vi "FTW-Example-SLASD-Add Actor.vi"(0 "FTW-Example-SLASD In":refnum<class "FTW-Example-SLASD.lvclass">, 11 "error in (no error)":errorcluster) -> (4 "FTW-Example-SLASD Out":refnum<class "FTW-Example-SLASD.lvclass">, 15 "error out":errorcluster)   [LabVIEW 2013, in "FTW-Example-SLASD.lvclass"]
uses:
  FTW-Example-SLASD.lvclass
  source/actor/Connector/FTW-ActorConnector.lvclass
panel:
  out "New Actor Inbox Address":string
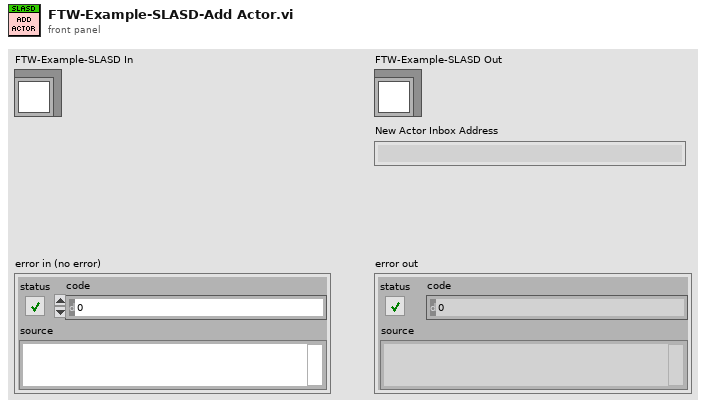
[diagram p1: front panel]
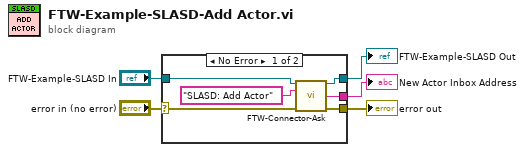
[diagram p0: block diagram]
diagram:
  n1 = case shown="No Error" "error in (no error)" {
    selector: "error in (no error)" -> [w9 w12]
    tunnel: "FTW-Example-SLASD In" -> [w11 w13]
    tunnel: [w10 w13] -> w3
    tunnel: [w8 w12] -> w2
    tunnel: [w6 _] -> w1
    frame No Error {
      n2 = call "FTW-Connector-Ask.vi"("FTW Actor Connector"=w11, "Request Header"="SLASD: Add Actor", "error in"=w9) -> ("FTW Actor Connector out"=w10:refnum<class "FTW-Example-SLASD.lvclass">, "Response Body"=w6:string, "error out"=w8:errorcluster)  [unwired: 7 in, 3 out]
    }
    frame Error {
    }
  }
  "FTW-Example-SLASD Out" <- w3
  "error out" <- w2
  "New Actor Inbox Address" <- w1
